vi "Frequency Mixer.vi"(8 "error in (no error)":errorcluster, 9 "Reference":T1, 10 "Signal []":waveform(dbl)[](array[waveform]), 11 "Lockin.DAQ":refnum<class "Instrument.DAQ.lvclass">) -> (0 "error out":errorcluster, 2 "Mixed":T1, 3 "Lockin.DAQ":refnum<class "Instrument.DAQ.lvclass">)   [LabVIEW 2019, in "Instrument.DAQ.lvclass"]
uses:
  Instrument.DAQ.lvclass
  Instrument.DAQ.lvclass/Instrument.DAQ.ctl
  <vilib>/measure/manoise.llb/Gaussian White Noise Waveform.vi
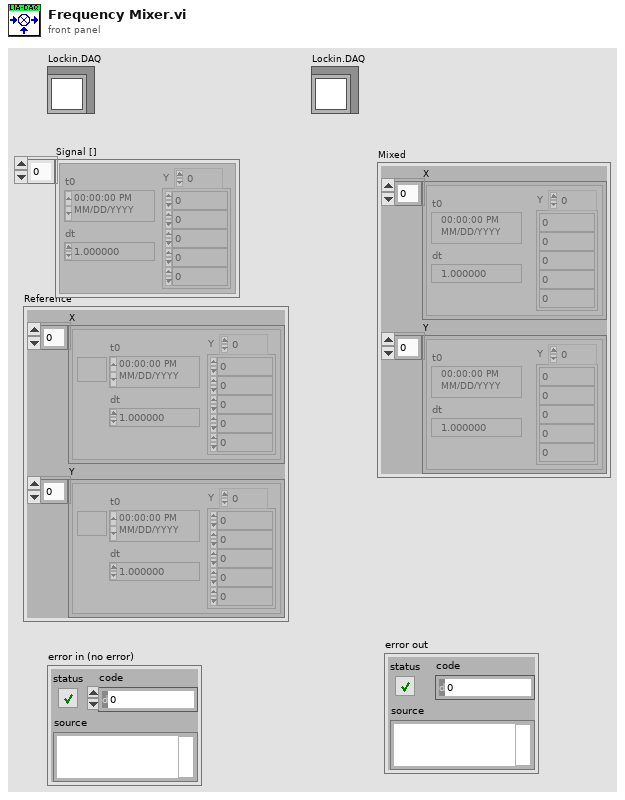
[diagram p1: front panel]
types:
  T1 = cluster{"X":waveform(dbl)[], "Y":waveform(dbl)[]}
  T2 = typedef "Instrument.DAQ.lvclass/AI-cluster.ctl" = T3[]
  T3 = typedef "Instrument UI.Lockin.lvclass/AI Channel--Cluster.ctl" = cluster{"Enable?":bool, "Channel":i32, "References":u16[]}
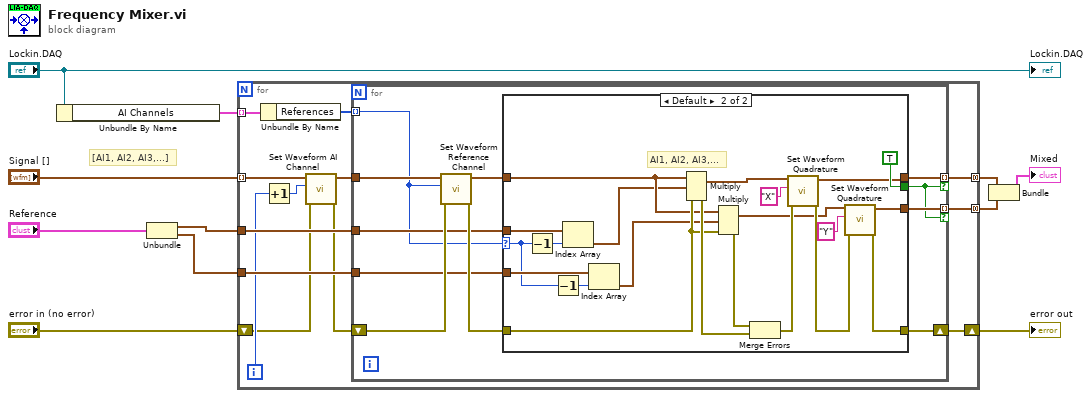
[diagram p0: block diagram]
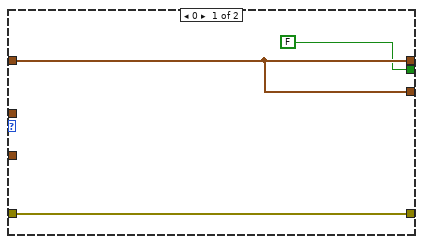
[diagram p2: hidden frame]
diagram:
  # "[AI1, AI2, AI3,...]"
  n1 = Unbundle By Name("Lockin.DAQ") -> ("AI Channels"=w7:T2)
  n2 = Unbundle("Reference") -> ("X"=w5:waveform(dbl)[], "Y"=w1:waveform(dbl)[])
  n3 = for {
    tunnel: [w21] -> w4 mode=concatenating
    tunnel: "Signal []" -> [w17] mode=indexing
    shift-right: [w24] -> w11
    shift-left: "error in (no error)" -> [w13]
    tunnel: w7 -> [w23] mode=indexing
    tunnel: w5 -> [w20]
    tunnel: w1 -> [w19]
    tunnel: [w18] -> w3 mode=concatenating
    i -> [w15]
    n4 = Unbundle By Name(w23) -> ("References"=w22:u16[])
    n5 = Increment(x=w15) -> (x+1=w14:i32)
    n6 = call "Set Waveform AI Channel.vi"("error in (no error)"=w13, "AI Channel"=w14, "Waveform in"=w17) -> ("error out"=w12:errorcluster, "Waveform out"=w16:waveform(dbl))  [unwired: 7 in]
    n7 = for {
      shift-right: [w35] -> w24
      shift-left: w12 -> [w33]
      tunnel: w22 -> [w26] mode=indexing
      tunnel: w16 -> [w27]
      tunnel: [w31] -> w21 mode=indexing if=w25
      tunnel: w20 -> [w30]
      tunnel: w19 -> [w29]
      tunnel: [w28] -> w18 mode=indexing if=w25
      n8 = call "Set Waveform Reference Channel.vi"("error in (no error)"=w33, "Reference Ch"=w26, "Waveform in"=w27) -> ("error out"=w32:errorcluster, "Waveform out"=w34:waveform(dbl))  [unwired: 7 in]
      n9 = case shown="Default" w26 {
        selector: w26 -> [_ w50]
        tunnel: [w38 w42] -> w35
        tunnel: w34 -> [w37 w55]
        tunnel: w32 -> [w38 w56]
        tunnel: [w37 w46] -> w31
        tunnel: [FALSE TRUE] -> w25
        tunnel: w30 -> [_ w53]
        tunnel: w29 -> [_ w51]
        tunnel: [w37 w45] -> w28
        frame 0 {
        }
        frame Default {
          # "AI1, AI2, AI3,..."
          n10 = Decrement(x=w50) -> (x-1=w59:u16)
          n11 = Decrement(x=w50) -> (x-1=w52:u16)
          n12 = Index Array(array=w53, index=w59) -> (element=w49:waveform(dbl))
          n13 = Index Array(array=w51, index=w52) -> (element=w48:waveform(dbl))
          n14 = Multiply(1:w49, 2:w55, 4:w56) -> (0:w47:waveform(dbl), 3:w57:errorcluster)
          n15 = Multiply(1:w48, 2:w55, 4:w56) -> (0:w41:waveform(dbl), 3:w58:errorcluster)
          n16 = Merge Errors(w58, w57) -> (w44:errorcluster)
          n17 = call "Set Waveform Quadrature.vi"("error in (no error)"=w44, "Quadratude"="X", "Waveform in"=w47) -> ("error out"=w43:errorcluster, "Waveform out"=w46:waveform(dbl))  [unwired: 7 in]
          n18 = call "Set Waveform Quadrature.vi"("error in (no error)"=w43, "Quadratude"="Y", "Waveform in"=w41) -> ("error out"=w42:errorcluster, "Waveform out"=w45:waveform(dbl))  [unwired: 7 in]
        }
      }
    }
  }
  "error out" <- w11
  n19 = Bundle(w4, w3) -> (→"Mixed":cluster{waveform(dbl)[], waveform(dbl)[]})  [unwired: 1 in]
  "Lockin.DAQ" <- "Lockin.DAQ"
